vi "Set Config.vi"(8 "error in (no error)":errorcluster, 9 "Config Data":variant, 11 "SimSyA in":refnum<class "SimSyA.lvclass">) -> (0 "error out":errorcluster, 3 "SimSyA out":refnum<class "SimSyA.lvclass">)   [LabVIEW 2014, in "SimSyA.lvlib" / "SimSyA.lvclass"]
uses:
  SimSyA.lvclass
  SimSyA.lvclass/SimSyA.ctl
  DriverMasterSync/build/DriverMasterSync.lvlibp/Modules/HAL/DriverMasterSync/DriverMasterSyncClass/DriverMasterSync.lvclass
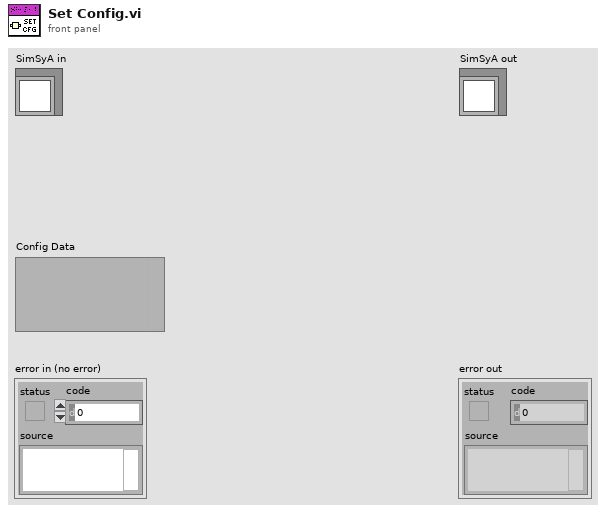
[diagram p1: front panel]
types:
  T1 = typedef "DriverMasterSync.lvlibp/HAL Config Data.ctl" = cluster{"HWSync Index":u32, "Driver Name":string, "Channel Mask":u64}
  T2 = cluster{"Channel Mask":u64, "DriverMasterSync out":refnum<class "SimSyA.lvclass">}
  T3 = cluster{"TDX":sgl[], "Encoder":i32, "DI Counter":u32, "DO Mask":u32}
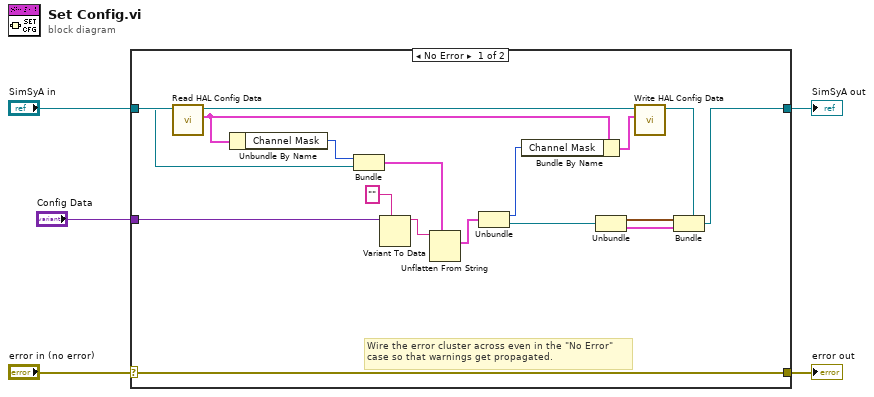
[diagram p0: block diagram]
diagram:
  n1 = case shown="No Error" "error in (no error)" {
    selector: "error in (no error)" -> [w22 w24]
    tunnel: [w22 w24] -> w4
    tunnel: [w10 w23] -> w2
    tunnel: "SimSyA in" -> [w20 w23]
    tunnel: "Config Data" -> [w21 _]
    frame No Error {
      # "Wire the error cluster across even in the \"No Error\"\ncase so that warnings get propagated."
      n2 = call "Read HAL Config Data.vi"("DriverMasterSync in"=w20) -> ("HAL Config Data"=w16:T1, "DriverMasterSync out"=w18:refnum<class "SimSyA.lvclass">)  [unwired: 8 in, 1 out]
      n3 = Unbundle By Name(w16) -> ("Channel Mask"=w17:u64)
      n4 = Bundle("Channel Mask"=w17, "DriverMasterSync out"=w18) -> (w7:T2)  [unwired: 1 in]
      n5 = Variant To Data(type="", Variant=w21) -> (data=w8:string)  [unwired: 1 in, 1 out]
      n6 = Unflatten From String(type=w7, binary string=w8) -> (value=w6:T2)  [unwired: 3 in, 2 out]
      n7 = Unbundle(w6) -> ("Channel Mask"=w15:u64, "DriverMasterSync out"=w19:refnum<class "SimSyA.lvclass">)
      n8 = Bundle By Name(cluster=w16, "Channel Mask"=w15) -> (w14:T1)
      n9 = Unbundle(w19) -> (w13:cluster{"Channel Mask":u64, "Max Seq Num":u64}, w12:T3)
      n10 = call "Write HAL Config Data.vi"("HAL Config Data"=w14, "DriverMasterSync in"=w18) -> ("DriverMasterSync out"=w11:refnum<class "SimSyA.lvclass">)  [unwired: 8 in, 1 out]
      n11 = Bundle(cluster=w11, w13, w12) -> (w10:refnum<class "SimSyA.lvclass">)
    }
    frame Error {
    }
  }
  "error out" <- w4
  "SimSyA out" <- w2
